vi "Polynomial Real Zeros Counter.vi"(9 "end":dbl format="%#.6g", 10 "start":dbl format="%#.6g", 11 "P(x)":dbl[](array[numeric])) -> (0 "error":i32, 3 "number of zeros":i32)   [LabVIEW 2020, in "NI_AALPro.lvlib"]
doc: "Calculates the number of zeros of the real polynomial <B>P(x)</B> in a real interval defined by <B>start</B> and <B>end</B> without determining the values of the zeros."
uses:
  NI_AALPro.lvlib
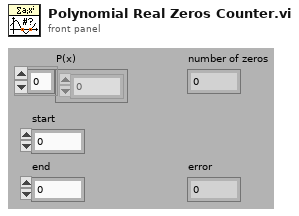
[diagram p1: front panel]
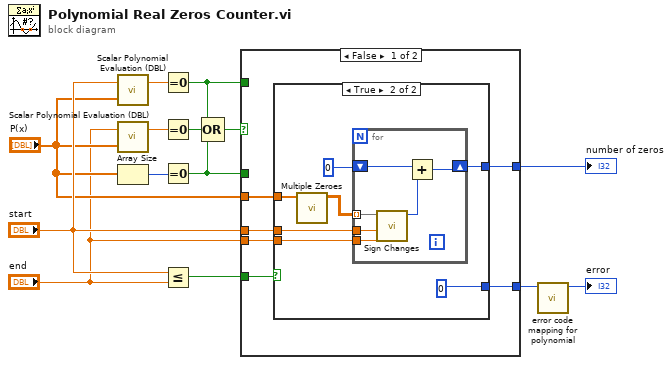
[diagram p0: block diagram]
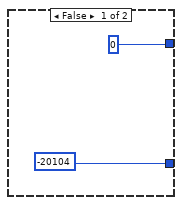
[diagram p2: hidden frame]
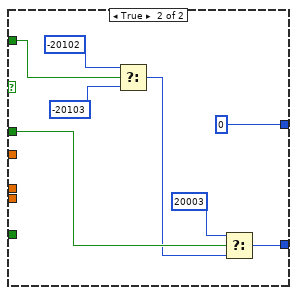
[diagram p3: hidden frame]
diagram:
  n1 = call "Scalar Polynomial Evaluation (DBL).vi"("P(x)"="P(x)", "a"="start") -> ("P(a)"=w6:dbl)  [unwired: 1 out]
  n2 = call "Scalar Polynomial Evaluation (DBL).vi"("P(x)"="P(x)", "a"="end") -> ("P(a)"=w3:dbl)  [unwired: 1 out]
  n3 = Array Size(array="P(x)") -> (size(s)=w12:i32)
  n4 = Equal To 0?(x=w6) -> (x = 0?=w10:bool)
  n5 = Equal To 0?(x=w3) -> (x = 0?=w11:bool)
  n6 = Equal To 0?(x=w12) -> (x = 0?=w8:bool)
  n7 = Less Or Equal?(x="start", y="end") -> (x <= y?=w13:bool)
  n8 = Compound Arithmetic op=OR(w10, w11, w8) -> (w9:bool)
  n9 = case shown="False" w9 {
    tunnel: [w20 w36] -> w2
    tunnel: "P(x)" -> [w19 _]
    tunnel: "start" -> [w18 _]
    tunnel: "end" -> [w17 _]
    tunnel: [w16 0 ("Numeric")] -> w14
    tunnel: w13 -> [w15 _]
    tunnel: w10 -> [_ w40]
    tunnel: w8 -> [_ w39]
    frame False {
      n10 = case shown="True" w15 {
        tunnel: [0 w29] -> w16
        tunnel: w17 -> [_ w28]
        tunnel: w18 -> [_ w27]
        tunnel: w19 -> [_ w24]
        tunnel: [-20104 ("start>end") 0] -> w20
        frame False {
        }
        frame True {
          n11 = call "Multiple Zeroes.vi"("p"=w24) -> ("sequence of polynomials"=w26:dbl[][])  [unwired: 10 in]
          n12 = for {
            shift-right: [w30] -> w29
            shift-left: 0 -> [w32]
            tunnel: w26 -> [w35] mode=indexing
            tunnel: w27 -> [w34]
            tunnel: w28 -> [w33]
            n13 = call "Sign Changes.vi"("x1"=w33, "x0"=w34, "f"=w35) -> ("number of roots"=w31:i32)  [unwired: 8 in]
            n14 = Add(x=w32, y=w31) -> (x+y=w30:i32)
          }
        }
      }
    }
    frame True {
      n15 = Select(t=-20102 ("start is root"), s=w40, f=-20103 ("end is root")) -> (s? t:f=w37:i32)
      n16 = Select(t=20003 ("empty array"), s=w39, f=w37) -> (s? t:f=w36:i32)
    }
  }
  "number of zeros" <- w14
  n17 = call "error code mapping for polynomial.vi"("error in"=w2) -> ("error out"=→"error":i32)  [unwired: 10 in]
